vi "Compile HHP.vi"(8 "error in (no error)":errorcluster, 10 "Help Path":path, 11 "temp .hhp path":path) -> (0 "error out":errorcluster, 1 "standard error":string, 2 "standard output":string)   [LabVIEW 2015, in "HTML Help File Tools.lvlib"]
uses:
  HTML Help File Tools.lvlib
  Log FGV Operation Modes.ctl
  Error Location.ctl
  <vilib>/regexp/Match Regular Expression.xnode
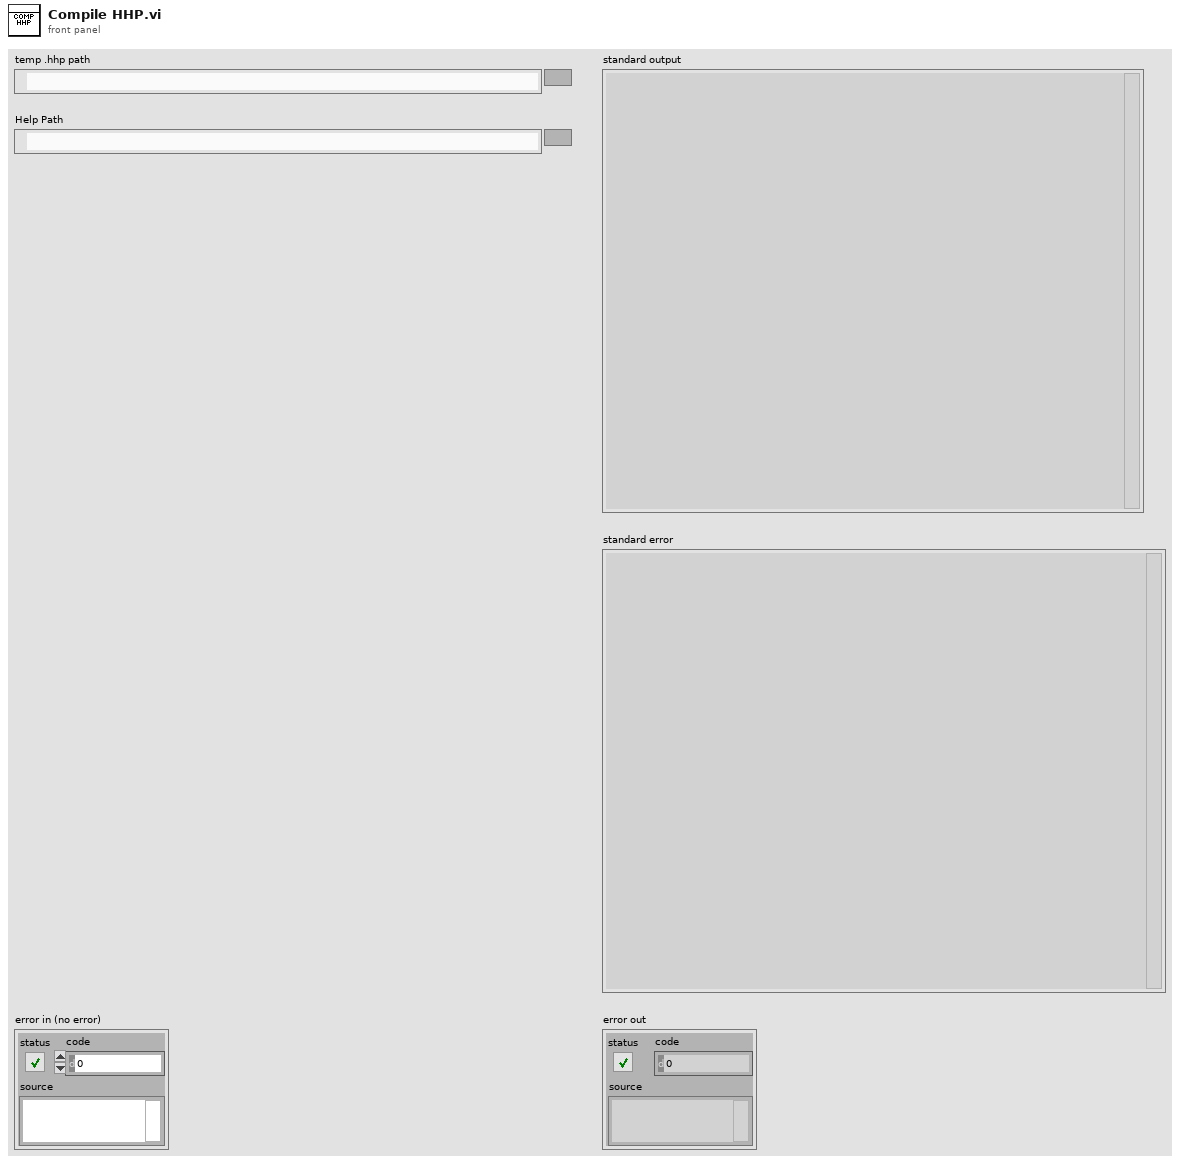
[diagram p1: front panel]
types:
  T1 = typedef "HTML Help File Tools.lvlib/Error Location.ctl" = enum16{"Delete tmp", "Compile HHP", "Find Install", "Create tmp", "Create HHP", "Find Help"}
  T2 = typedef "HTML Help File Tools.lvlib/Log FGV Operation Modes.ctl" = enum16{"Close", "Write", "Open File"}
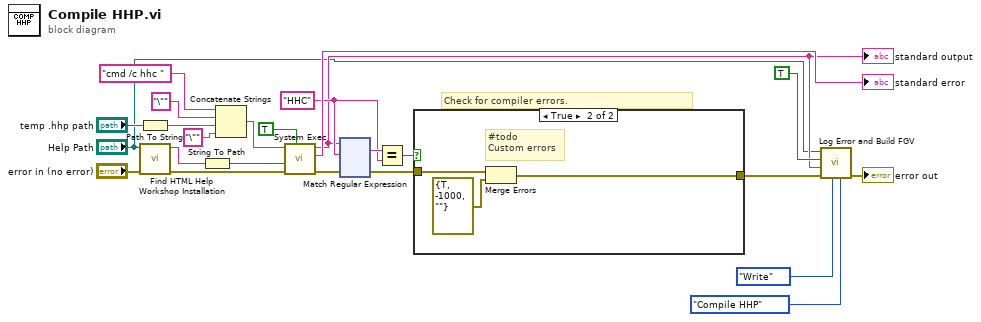
[diagram p0: block diagram]
diagram:
  w7 = "HHC" ("regular expression")
  # "Check for compiler errors."
  n1 = Path To String(path="temp .hhp path") -> (string=w22:string)
  n2 = call "Find HTML Help Workshop Installation.vi"("error in (no error)"="error in (no error)", "Help Path"="Help Path") -> ("error out"=w16:errorcluster, "Installation Path"=w15:string)  [unwired: 8 in]
  n3 = String To Path(string=w15) -> (path=w14:path)
  n4 = Concatenate Strings("cmd /c hhc " ("string"), "\"" ("string"), w22, "\"" ("string")) -> (w18:string)
  n5 = call <vilib>:"System Exec.vi"("wait until completion? (T)"=TRUE, "error in (no error)"=w16, "working directory"=w14, "command line"=w18) -> ("error out"=w4:errorcluster, "standard error"=→"standard error":string, "standard output"=w2:string)  [unwired: 4 in, 1 out]
  "standard output" <- w2
  n6 = xnode "Match Regular Expression"("input string"=w2, "regular expression"=w7, "error in"=w4) -> ("whole match"=w8:string, "error out"=w5:errorcluster)  [unwired: 3 in, 3 out]
  n7 = Equal?(x=w8, y=w7) -> (x = y?=w6:bool)
  n8 = case shown="True" w6 {
    tunnel: [w25 w28] -> w3
    tunnel: w5 -> [w25 w27]
    frame False {
    }
    frame True {
      # "#todo\nCustom errors"
      n9 = Merge Errors(w27, errorcluster {"status"=TRUE, "code"=-1000, "source"=""} ("error constant")) -> (w28:errorcluster)
    }
  }
  n10 = call "Log Error and Build FGV.vi"("Error Location"=Error_Location."Compile HHP", "Operation Mode"=Log_FGV_Operation_Modes."Write", "error in"=w3, "Build Output"=w2, "Log Build Output?"=TRUE, "Help Documentation Path"="Help Path") -> ("error out"=→"error out":errorcluster)  [unwired: 5 in]
